vi "Rearrange_Binary.vi"(8 "error in (no error)":errorcluster, 11 "String in":string) -> (0 "error out":errorcluster, 3 "String out":string)   [LabVIEW 2016]
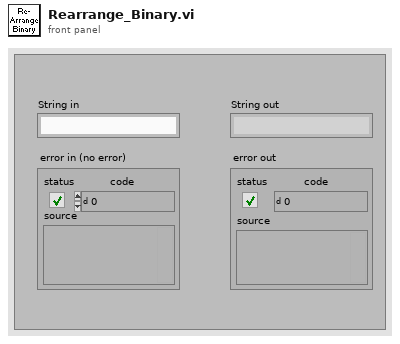
[diagram p1: front panel]
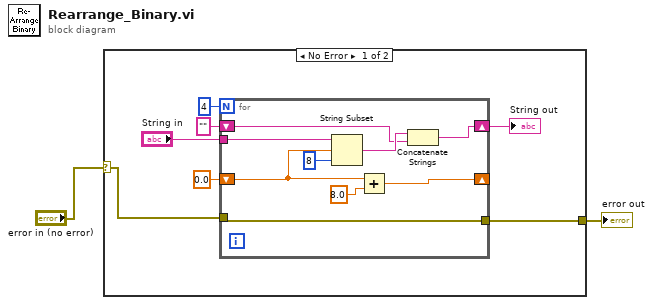
[diagram p0: block diagram]
diagram:
  n1 = case shown="No Error" "error in (no error)" {
    selector: "error in (no error)" -> [w3 w19]
    tunnel: [w5 w19] -> w2
    frame No Error {
      n2 = for {
        N: 4 -> [_]
        tunnel: "String in" -> [w18]
        shift-right: [w13] -> w8
        shift-left: "" -> [w11]
        shift-right: [w15] -> _
        shift-left: 0.0 -> [w14]
        tunnel: w3 -> [w10]
        tunnel: [w10] -> w5
        n3 = String Subset(string=w18, offset (0)=w14, length (rest)=8 ("length (rest)")) -> (substring=w12:string)
        n4 = Add(x=w14, y=8.0) -> (x+y=w15:dbl)
        n5 = Concatenate Strings(w12, w11) -> (w13:string)
      }
      "String out" <- w8
    }
    frame Error {
    }
  }
  "error out" <- w2
